vi "Calculate_Rotation_Tomography_v1.vi"(0 "Diff signal":T1, 5 "Sum signal":T1, 7 "Monitor to RF ratio":dbl=-27.79, 11 "Summed data in":T1) -> (4 "rotation signal":cluster{"Time":dbl[], dbl[]}[](array[cluster]), 6 "rotation spectrum":waveform(dbl)[](array[waveform]), 8 "differ signal":cluster{"Time":dbl[], "Y":dbl[]}[](array[cluster]), 10 "absorption signal":cluster{"Time":dbl[], dbl[]}, 13 "Imbalance X/Y":dbl[](array[numeric]), 15 "Summed data out":T1)   [LabVIEW 2021]
uses:
  Ver_1/Cutted_Data.ctl
  <vilib>/Analysis/baseanly.llb/Mean (DBL).vi
  <vilib>/Analysis/NI_AALPro.lvlib
  <vilib>/Analysis/NI_AALBase.lvlib
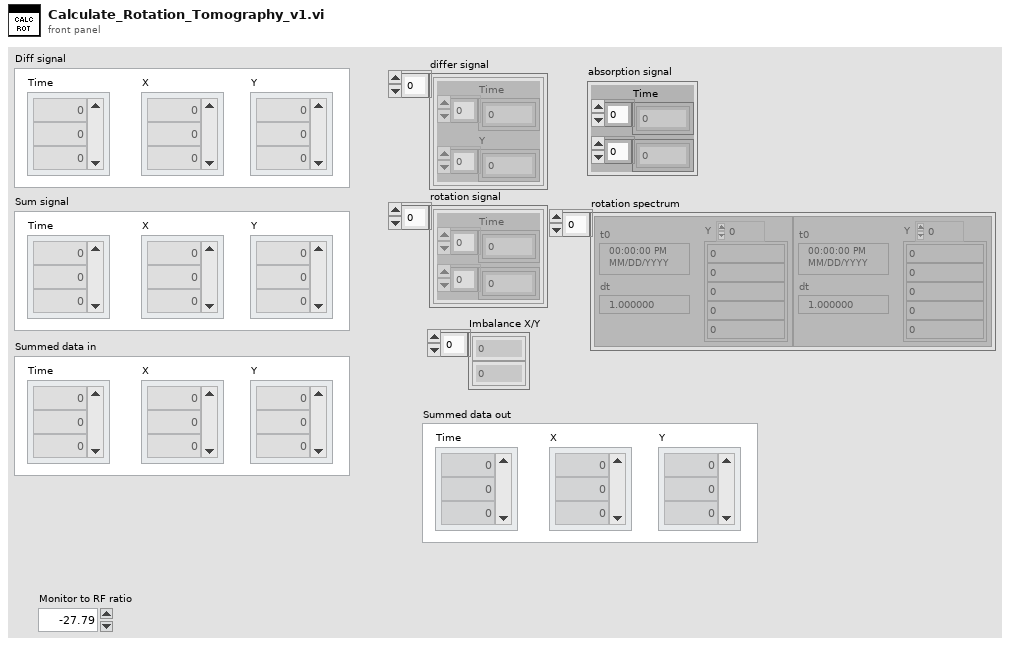
[diagram p1: front panel]
types:
  T1 = typedef "Cutted_Data.ctl" = cluster{"X":dbl[], "Y":dbl[], "Time":dbl[]}
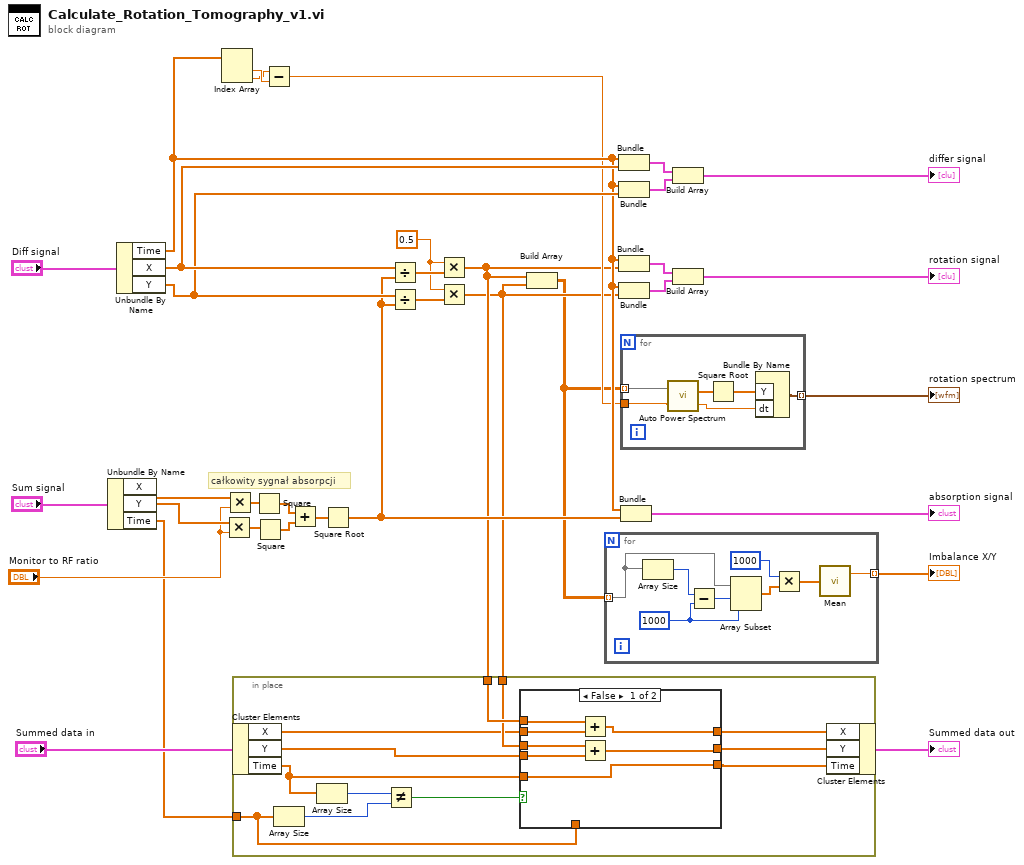
[diagram p0: block diagram]
diagram:
  w23 = 0.5
  # "całkowity sygnał absorpcji"
  n1 = Unbundle By Name("Sum signal") -> ("X"=w33:dbl[], "Y"=w32:dbl[], "Time"=w8:dbl[])
  n2 = Unbundle By Name("Diff signal") -> ("Time"=w12:dbl[], "X"=w20:dbl[], "Y"=w19:dbl[])
  n3 = Index Array(array=w12) -> (element #1=w2:dbl, element #2=w1:dbl)  [unwired: 2 in]
  n4 = Multiply(x=w32, y="Monitor to RF ratio") -> (x*y=w29:dbl[])
  n5 = Multiply(x=w33, y="Monitor to RF ratio") -> (x*y=w30:dbl[])
  n6 = Square(x=w30) -> (x^2=w28:dbl[])
  n7 = Square(x=w29) -> (x^2=w27:dbl[])
  n8 = Subtract(x=w1, y=w2) -> (x-y=w11:dbl)
  n9 = Add(x=w28, y=w27) -> (x+y=w26:dbl[])
  n10 = Square Root(x=w26) -> (sqrt(x)=w14:dbl[])
  n11 = Divide(x=w20, y=w14) -> (x/y=w24:dbl[])
  n12 = Divide(x=w19, y=w14) -> (x/y=w25:dbl[])
  n13 = Multiply(x=w23, y=w24) -> (x*y=w7:dbl[])
  n14 = Multiply(x=w23, y=w25) -> (x*y=w6:dbl[])
  n15 = in-place {
    in-place-border: w8 -> [w37]
    in-place-border: w7 -> [w42]
    in-place-border: w6 -> [w41]
    n16 = in-place-cluster #1("Summed data in") -> ("X"=w40:dbl[], "Y"=w39:dbl[], "Time"=w38:dbl[])
    n17 = Array Size(array=w37) -> (size(s)=w45:i32)
    n18 = Array Size(array=w38) -> (size(s)=w47:i32)
    n19 = Not Equal?(x=w47, y=w45) -> (x != y?=w46:bool)
    n20 = case shown="False" w46 {
      tunnel: [w49 w56] -> w44
      tunnel: [w52 w57] -> w43
      tunnel: w42 -> [w53 w57]
      tunnel: w41 -> [w51 w56]
      tunnel: w40 -> [w54 _]
      tunnel: w39 -> [w50 _]
      tunnel: w38 -> [w48 _]
      tunnel: [w48 w55] -> w36
      tunnel: w37 -> [_ w55]
      frame False {
        n21 = Add(x=w53, y=w54) -> (x+y=w52:dbl[])
        n22 = Add(x=w51, y=w50) -> (x+y=w49:dbl[])
      }
      frame True {
      }
    }
    n23 = in-place-cluster #1("X"=w43, "Y"=w44, "Time"=w36) -> (→"Summed data out":T1)
  }
  n24 = Build Array(w7, w6) -> (w4:dbl[][])
  n25 = for {
    tunnel: w4 -> [w62] mode=indexing
    tunnel: [w59] -> w3 mode=indexing
    w63 = 1000
    n26 = Array Size(array=w62) -> (size(s)=w65:i32)
    n27 = Subtract(x=w65, y=w63) -> (x-y=w64:i32)
    n28 = Array Subset(array=w62, index=w64, length=w63) -> (w61:dbl[])
    n29 = Multiply(x=1000, y=w61) -> (x*y=w58:dbl[])
    n30 = call-poly <vilib>:"Mean.vi"("X"=w58) -> ("mean"=w59:dbl)  [unwired: 1 out]
  }
  "Imbalance X/Y" <- w3
  n31 = Bundle("Time"=w12, "X"=w20) -> (w22:cluster{"Time":dbl[], "X":dbl[]})  [unwired: 1 in]
  n32 = Bundle("Time"=w12, "Y"=w19) -> (w21:cluster{"Time":dbl[], "Y":dbl[]})  [unwired: 1 in]
  n33 = Bundle("Time"=w12, w7) -> (w16:cluster{"Time":dbl[], dbl[]})  [unwired: 1 in]
  n34 = Bundle("Time"=w12, w6) -> (w17:cluster{"Time":dbl[], dbl[]})  [unwired: 1 in]
  n35 = for {
    tunnel: w4 -> [w71] mode=indexing
    tunnel: w11 -> [w70]
    tunnel: [w66] -> w10 mode=indexing
    n36 = call <vilib>:"Auto Power Spectrum.vi"("dt"=w70, "Signal (V)"=w71) -> ("df"=w67:dbl, "Power Spectrum (V^2 rms)"=w69:dbl[])
    n37 = Square Root(x=w69) -> (sqrt(x)=w68:dbl[])
    n38 = Bundle By Name("Y"=w68, "dt"=w67) -> (w66:waveform(dbl))  [unwired: 1 in]
  }
  "rotation spectrum" <- w10
  n39 = Bundle("Time"=w12, w14) -> (→"absorption signal":cluster{"Time":dbl[], dbl[]})  [unwired: 1 in]
  n40 = Build Array(w22, w21) -> (→"differ signal":cluster{"Time":dbl[], "Y":dbl[]}[])
  n41 = Build Array(w16, w17) -> (→"rotation signal":cluster{"Time":dbl[], dbl[]}[])
